vi "Optics_SetVelocity.VI"(8 "Error in":errorcluster, 9 "Velocity":dbl, 10 "Motor":dbl, 11 "VISA in":refnum<visa-resource-name>) -> (0 "Error out":errorcluster, 3 "VISA out":refnum<visa-resource-name>)   [LabVIEW 2021]
panel:
  out "String sent":string
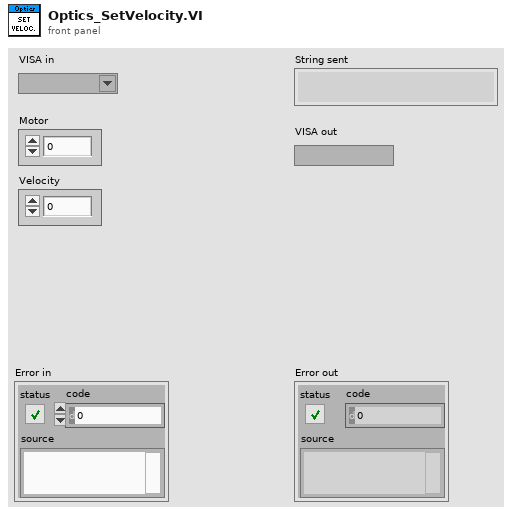
[diagram p1: front panel]
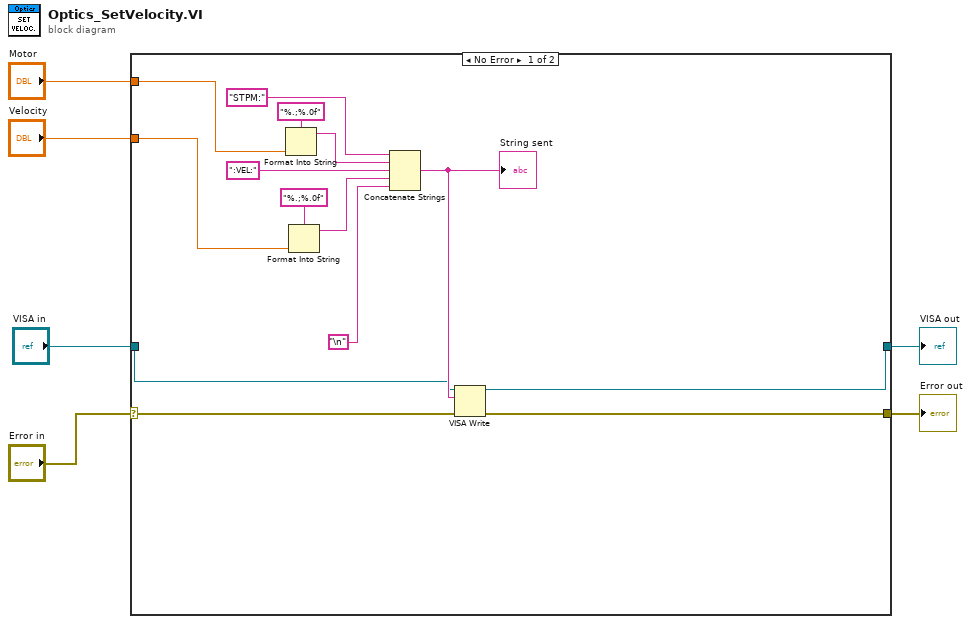
[diagram p0: block diagram]
diagram:
  n1 = case shown="No Error" "Error in" {
    selector: "Error in" -> [w9 w22]
    tunnel: [w8 w22] -> w6
    tunnel: "Motor" -> [w17 _]
    tunnel: "VISA in" -> [w10 w21]
    tunnel: "Velocity" -> [w16 _]
    tunnel: [w7 w21] -> w1
    frame No Error {
      n2 = Format Into String(format string="%.;%.0f", w17) -> (resulting string=w20:string)  [unwired: 2 in, 1 out]
      n3 = Format Into String(format string="%.;%.0f", w16) -> (resulting string=w15:string)  [unwired: 2 in, 1 out]
      n4 = Concatenate Strings("STPM:", w20, ":VEL:", w15, "\n") -> (w11:string)
      "String sent" <- w11
      n5 = VISA Write(VISA resource name=w10, write buffer=w11, error in (no error)=w9) -> (VISA resource name out=w7:refnum<visa-resource-name>, error out=w8:errorcluster)  [unwired: 1 out]
    }
    frame Default {
    }
  }
  "Error out" <- w6
  "VISA out" <- w1
